vi "WaveformCharGlobal.vi"() -> ()   [LabVIEW 2018]
panel:
  out "Waveform Chart":dbl(graph)
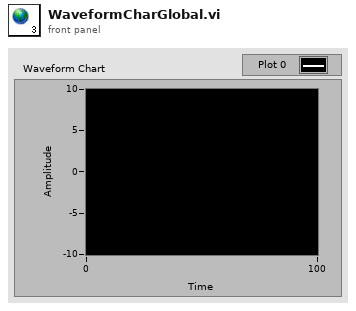
[diagram p1: front panel]
diagram:
